vi "Simple Scripting Example - Add on Python Side.vi"() -> ()   [LabVIEW 2013]
uses:
  LabVIEW Core/TS.lvlib
  LabVIEW Core/LabVIEW Python Connector Message.ctl
panel:
  out "error out":errorcluster
  out "Sum":string
  in  "Numbers to Add":dbl[](array[numeric])
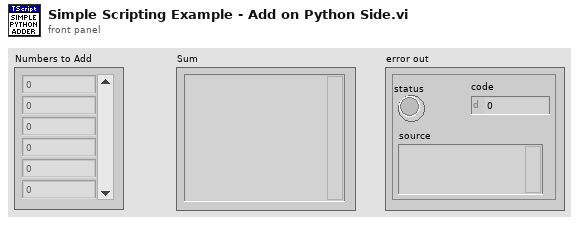
[diagram p1: front panel]
types:
  T1 = typedef "TS.lvlib/LabVIEW Python Connector Message.ctl" = cluster{"Command":string, "Data":string[], "Script ID":i64, "LabVIEW Server ID":string, "Python Message ID":i32}
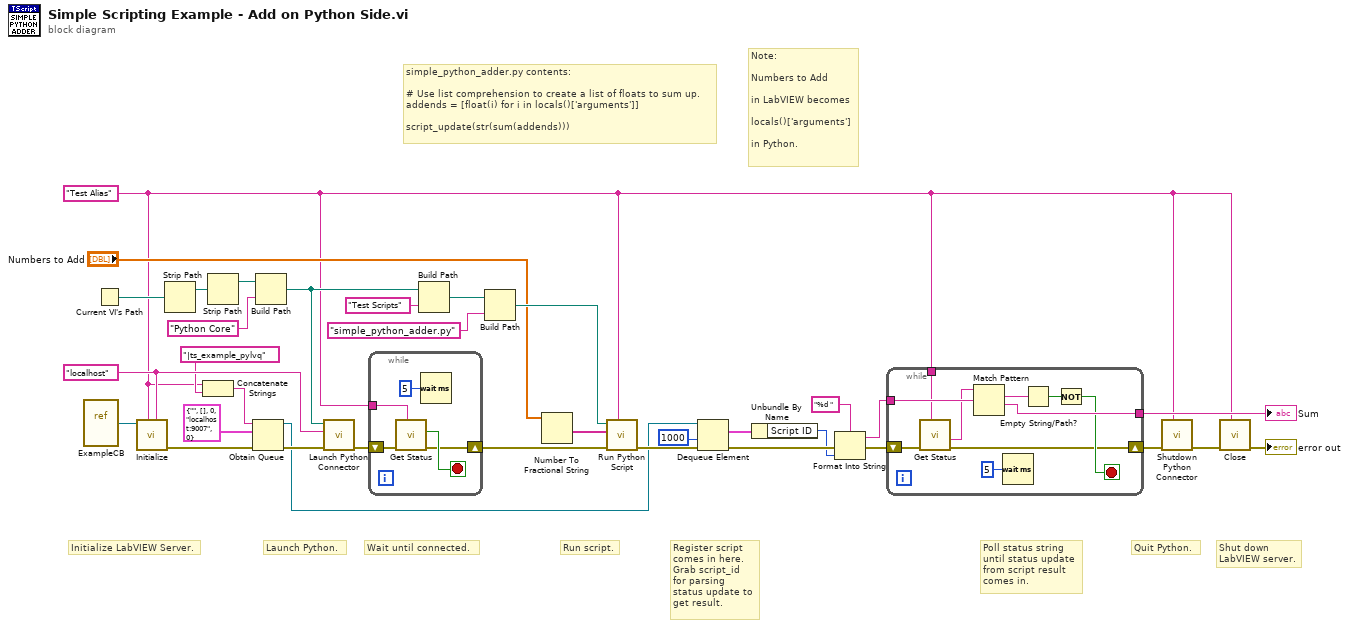
[diagram p0: block diagram]
diagram:
  w1 = "Test Alias" ("IP Address for LabVIEW Server")
  w26 = "localhost" ("IP Address for LabVIEW Server")
  # "Note: \n\nNumbers to Add\n\nin LabVIEW becomes\n\nlocals()['arguments']\n\nin Python."
  # "simple_python_adder.py contents:\n\n# Use list comprehension to create a list of floats to sum up.\naddends = [float(i) for i in locals()['arguments']]\n\nscript_update(str(sum(addends)))"
  # "Shut down\nLabVIEW server."
  # "Quit Python."
  # "Poll status string\nuntil status update\nfrom script result\ncomes in."
  # "Register script\ncomes in here.\nGrab script_id\nfor parsing\nstatus update to\nget result."
  # "Run script."
  # "Wait until connected."
  # "Launch Python."
  # "Initialize LabVIEW Server."
  n1 = vi-ref "ExampleCB.vi"() -> (w34:refnum<vi>)
  n2 = Current VI's Path() -> (path=w27:path)
  n3 = call "Initialize.vi"("IP Address for LabVIEW Server"=w26, "Server Alias"=w1, "VI Refnum"=w34) -> ("error out"=w32:errorcluster)  [unwired: 8 in]
  n4 = Strip Path(path=w27) -> (stripped path=w29:path)  [unwired: 1 out]
  n5 = Concatenate Strings(w1, "|ts_example_pylvq" ("name (unnamed)")) -> (w2:string)
  n6 = Strip Path(path=w29) -> (stripped path=w30:path)  [unwired: 1 out]
  n7 = Obtain Queue(name (unnamed)=w2, element data type=T1 {"Command"="", "Data"=[], "Script ID"=0, "LabVIEW Server ID"="localhost:9007", "Python Message ID"=0} ("element"), error in (no error)=w32) -> (queue out=w17:refnum<queue>, error out=w31:errorcluster)  [unwired: 2 in, 1 out]
  n8 = Build Path(base path=w30, name or relative path="Python Core") -> (appended path=w25:path)
  n9 = call "Launch Python Connector.vi"("error in (no error)"=w31, "Tell Python the IP Address Where LabVIEW Is"=w26, "Path to Python Core Folder"=w25) -> ("error out"=w20:errorcluster)  [unwired: 8 in]
  n10 = while {
    shift-right: [w37] -> w19
    shift-left: w20 -> [w39]
    tunnel: w1 -> [w35]
    stop <- w38 stop-if-true
    n11 = call "Get Status.vi"("Server Alias"=w35, "error in (no error)"=w39) -> ("error out"=w37:errorcluster, "Connected"=w38:bool)  [unwired: 4 in, 4 out]
    n12 = Wait (ms)(milliseconds to wait=u32 5) -> ()  [unwired: 1 out]
  }
  n13 = Build Path(base path=w25, name or relative path="Test Scripts") -> (appended path=w23:path)
  n14 = Build Path(base path=w23, name or relative path="simple_python_adder.py") -> (appended path=w21:path)
  n15 = Number To Fractional String(number="Numbers to Add") -> (F-format string=w4:string[])  [unwired: 3 in]
  n16 = call "Run Python Script.vi"("Server Alias"=w1, "error in (no error)"=w19, "Script Arguments (Optional)"=w4, "Absolute Python Script Path"=w21) -> ("error out"=w18:errorcluster)  [unwired: 7 in]
  n17 = Dequeue Element(queue=w17, timeout in ms (-1)=1000, error in (no error)=w18) -> (element=w15:T1, error out=w14:errorcluster)  [unwired: 2 out]
  n18 = Unbundle By Name(w15) -> ("Script ID"=w13:i64)
  n19 = Format Into String(format string="%d ", error in=w14, w13) -> (resulting string=w11:string, error out=w12:errorcluster)  [unwired: 1 in]
  n20 = while {
    shift-right: [w42] -> w7
    shift-left: w12 -> [w49]
    tunnel: w11 -> [w48]
    tunnel: [w45] -> w9
    tunnel: w1 -> [w40]
    stop <- w43 stop-if-true
    n21 = call "Get Status.vi"("Server Alias"=w40, "error in (no error)"=w49) -> ("error out"=w42:errorcluster, "Script Status"=w47:string)  [unwired: 4 in, 4 out]
    n22 = Match Pattern(string=w47, regular expression=w48) -> (match substring=w46:string, after substring=w45:string)  [unwired: 1 in, 2 out]
    n23 = Wait (ms)(milliseconds to wait=u32 5) -> ()  [unwired: 1 out]
    n24 = Empty String/Path?(string/path=w46) -> (empty?=w44:bool)
    n25 = Not(x=w44) -> (.not. x?=w43:bool)
  }
  "Sum" <- w9
  n26 = call "Shutdown Python Connector.vi"("Server Alias"=w1, "error in (no error)"=w7) -> ("error out"=w8:errorcluster)  [unwired: 9 in]
  n27 = call "Close.vi"("Server Alias"=w1, "error in (no error)"=w8) -> ("error out"=→"error out":errorcluster)  [unwired: 9 in]
